vi "Handle Endianity.vi"(8 "error in (no error)":errorcluster, 10 "Byte to read in":string, 11 "TCP Listener in":refnum<class "TCP Listener.lvclass">) -> (0 "error out":errorcluster, 2 "Bytes to read out":string, 3 "TCP Listener out":refnum<class "TCP Listener.lvclass">)   [LabVIEW 2026, in "TALOS.lvlib" / "TCP Listener.lvlib" / "TCP Listener.lvclass"]
uses:
  TCP Listener.lvclass
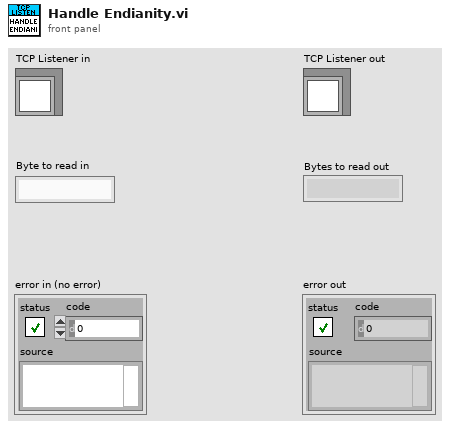
[diagram p1: front panel]
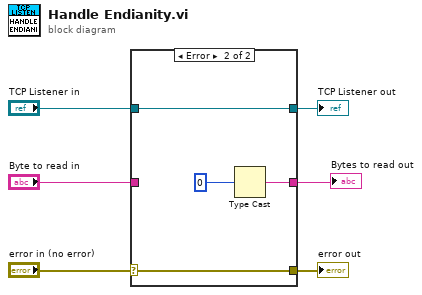
[diagram p0: block diagram]
diagram:
  n1 = case shown="Error" "error in (no error)" {
    selector: "error in (no error)" -> [w8 w13]
    tunnel: [w8 w13] -> w5
    tunnel: [w9 w12] -> w3
    tunnel: "TCP Listener in" -> [w9 w12]
    tunnel: "Byte to read in" -> [w7 _]
    tunnel: [w7 w11] -> w1
    frame No Error {
    }
    frame Error {
      n2 = Type Cast(x=0) -> (*(type *) &x=w11:string)  [unwired: 1 in]
    }
  }
  "error out" <- w5
  "TCP Listener out" <- w3
  "Bytes to read out" <- w1
